vi "FGV Externe Stickstoff Befuellung.vi"(8 "Aktion":T2=enum."Befüllen vorbereiten", 11 "Stiskstoff Befüllzeiten":T1) -> (0 "Ausgang":bool, 1 "Befülldauer":sgl, 2 "Befüllen 2":timestamp, 3 "Befüllen 1":timestamp, 4 "Befüllzeit":dbl, 5 "Timeout":bool, 6 "Aktion":T2=enum."Befüllen vorbereiten")   [LabVIEW 2020, in "Externe Stickstoff Befuellung.lvlib"]
uses:
  Externe Stickstoff Befuellung.lvlib
  Aktionen Externe Stockstoff Befuellung.ctl
  Externe Stickstoff Befuellzeiten.ctl
  Verwaltung/FGV IN Aktionen.ctl
  Konfig-Dateien/FGV Betriebsdaten Aktionen.ctl
  Allgemein/Allgemein.lvlib
  Konfig-Dateien/Konfig-Dateien.lvlib
  Verwaltung/Verwaltung - cRIO.lvlib
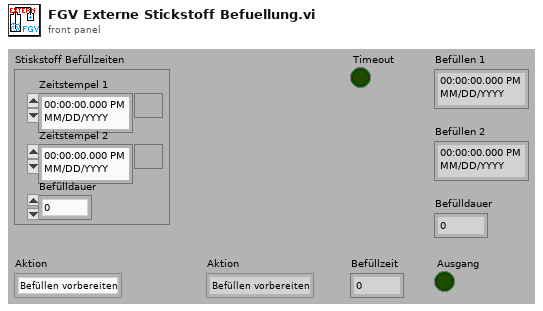
[diagram p1: front panel]
types:
  T1 = typedef "Externe Stickstoff Befuellung.lvlib/Externe Stickstoff Befuellzeiten.ctl" = cluster{"Zeitstempel 1":timestamp, "Zeitstempel 2":timestamp, "Befülldauer":sgl}
  T2 = typedef "Externe Stickstoff Befuellung.lvlib/Aktionen Externe Stockstoff Befuellung.ctl" = enum16{"lesen", "Befüllen vorbereiten", "Befüllen", "Befüllen beenden", "Warten", "deaktiviert", "initialisieren"}
  T3 = typedef "Verwaltung - cRIO.lvlib/FGV IN Aktionen.ctl" = enum16{"lesen", "DI", "AI", "Fühler Br.", "TC", "Fühler Br. TC"}
  T4 = typedef "Konfig-Dateien.lvlib/FGV Betriebsdaten Aktionen.ctl" = enum16{"lesen", "Anlagengrenzw.", "PID Param.", "Sonstige", "Sensor Para."}
  T5 = typedef "Verwaltung - cRIO.lvlib/Digital Eingaenge 0-15.ctl" = cluster{"I0: N2 Nachf. FT-IR voll":bool, "I1: N2 Nachf. Vorrat leer":bool, "I2: (Klimaanlage eingeschaltet)":bool, "I3: (Klimaanlage Störung)":bool, "I4: Trigger Eingang (Messdaten sp.)":bool, "I5: Reserve":bool, "I6: Reserve":bool, "I7: Reserve":bool, "I8: Druckschalter Versorgung ok":bool, "I9: Reserve":bool, "I10: Reserve":bool, "I11: Reserve":bool, "I12: Drucksch. N2 Versorgung":bool, "I13: Reserve":bool, "I14: Drucksch. N2 Optikbox":bool, "I15: (Füllstand Kondensatbehälter)":bool}
  T6 = typedef "Erweiterte Konfig.lvlib/Sonstige Parameter.ctl" = cluster{"Lüfter langsam":sgl, "Lüfter schnell":sgl, "FT-IR Kühlung Soll":sgl, "FT-IR Kühlung Max":sgl, "Überwachung":T7, "Befüllung aktiv":T8, "Stickstoff Befüllzeit":sgl, "Befüllintervall":sgl, "Kalibrierwert FT-IR":sgl, "Offset Ausgang":sgl, "Offset FT-IR":sgl, "Offset Druck FT-IR":sgl, "Dichtheitstest Zeit":sgl, "Dichtheitstest Abfall":sgl, "Dichtheitstest Umfang":T9, "Offset Umgebung":sgl, "Max Taupunkt":sgl, "Pumpendrehzahl":sgl, "ext. Befüllung":T8, "Ext. Stickstoff Befüllzeit":sgl}
  T7 = typedef "Auswahlfeld.ctl" = u16
  T8 = typedef "LogKonfig.lvlib/Auswahlfeld aktiviert-deaktiviert.ctl" = u16
  T9 = typedef "Erweiterte Konfig.lvlib/Dichtheitstest Umfang.ctl" = u16
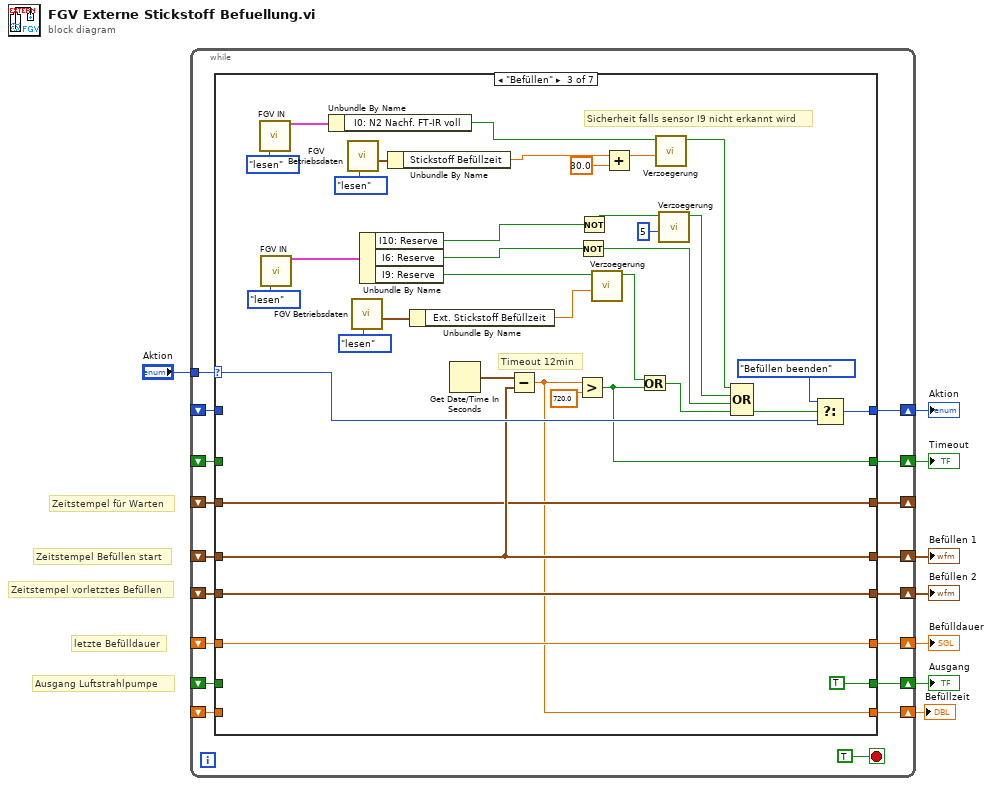
[diagram p0: block diagram]
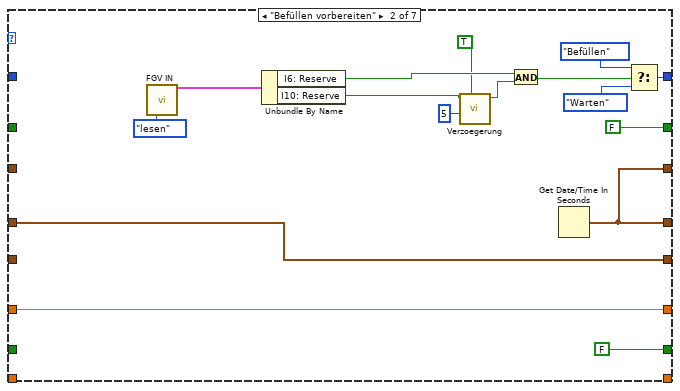
[diagram p3: hidden frame]
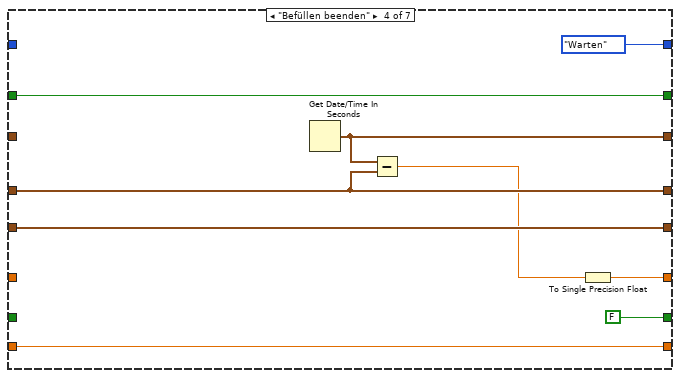
[diagram p4: hidden frame]
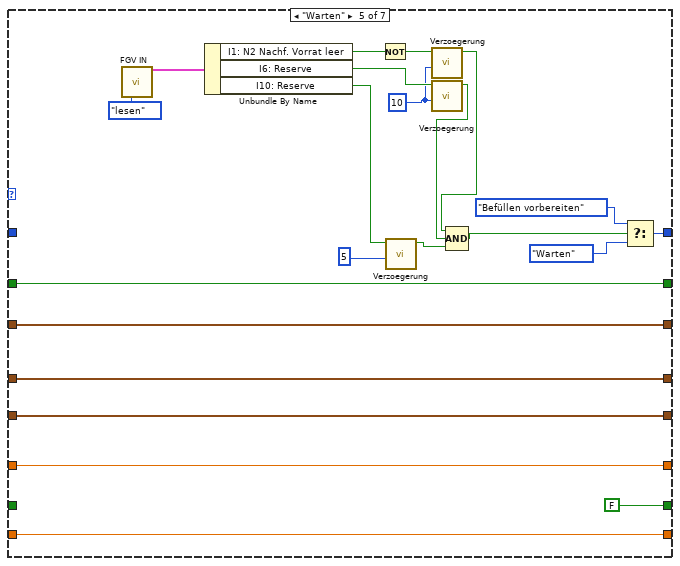
[diagram p5: hidden frame]
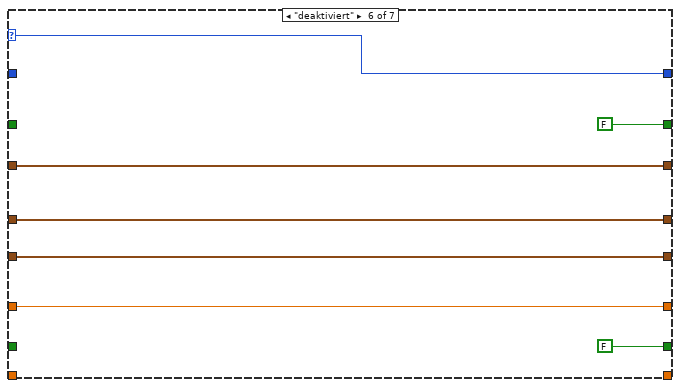
[diagram p6: hidden frame]
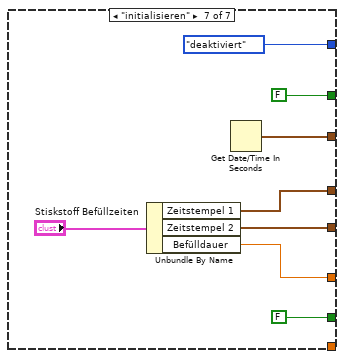
[diagram p7: hidden frame]
diagram:
  # "Zeitstempel für Warten"
  # "Ausgang Luftstrahlpumpe"
  # "Zeitstempel vorletztes Befüllen"
  # "letzte Befülldauer"
  # "Zeitstempel Befüllen start"
  n1 = while {
    tunnel: "Aktion" -> [w23]
    shift-right: [w20] -> w7
    shift-left: _ -> [w18]
    shift-right: [w24] -> w5
    shift-left: _ -> [w16]
    shift-right: [w19] -> w6
    shift-left: _ -> [w17]
    shift-right: [w25] -> w4
    shift-left: _ -> [w15]
    shift-right: [w21] -> w8
    shift-left: _ -> [w14]
    shift-right: [w22] -> w3
    shift-left: _ -> [w13]
    shift-right: [w11] -> _
    shift-left: _ -> [w12]
    shift-right: [w10] -> w1
    shift-left: _ -> [w9]
    stop <- TRUE stop-if-true
    n2 = case shown="\"Befüllen\"" w23 {
      selector: w23 -> [_ _ w84 _ _ w124 _]
      tunnel: [w29 w40 w77 Aktionen_Externe_Stockstoff_Befuellung."Warten" ("Aktion") w111 w124 Aktionen_Externe_Stockstoff_Befuellung."deaktiviert" ("Aktion")] -> w22
      tunnel: [w34 w46 w80 w93 w115 w122 w130] -> w20
      tunnel: [w31 FALSE TRUE FALSE FALSE FALSE FALSE] -> w25
      tunnel: w18 -> [w34 w49 w80 w93 w115 w122 _]
      tunnel: [w32 w48 w81 w88 w112 w120 w131] -> w24
      tunnel: w16 -> [w32 w48 w81 _ w112 w120 _]
      tunnel: [w33 w49 w82 w94 w116 w121 w129] -> w19
      tunnel: w17 -> [w33 _ w82 w94 w116 w121 _]
      tunnel: w15 -> [w31 _ _ _ _ _ _]
      tunnel: [w30 FALSE w74 w91 w109 FALSE FALSE] -> w21
      tunnel: w14 -> [w30 _ _ w91 w109 _ _]
      tunnel: w13 -> [w29 _ _ _ _ _ _]
      tunnel: w12 -> [w28 _ w73 _ w110 w118 _]
      tunnel: [w28 w46 w73 w90 w110 w118 w125] -> w11
      tunnel: [w27 _ w64 w87 w100 _ _] -> w10
      tunnel: w9 -> [w27 _ _ w87 w100 _ _]
      frame "lesen", Default {
      }
      frame "Befüllen vorbereiten" {
        n3 = call "FGV IN.vi"("Aktion"=FGV_IN_Aktionen."lesen") -> ("DI"=w45:T5)  [unwired: 10 in, 4 out]
        n4 = Unbundle By Name(w45) -> ("I6: Reserve"=w41:bool, "I10: Reserve"=w38:bool)
        n5 = call "Verzoegerung.vi"("Abfallverzögerung?"=TRUE, "sec"=u16 5, "Startsignal"=w38) -> ("Zeit abgelaufen?"=w35:bool)  [unwired: 7 in, 1 out]
        n6 = And(x=w41, y=w35) -> (x .and. y?=w39:bool)
        n7 = Get Date/Time In Seconds() -> (seconds since 1Jan1904=w46:timestamp)
        n8 = Select(t=Aktionen_Externe_Stockstoff_Befuellung."Befüllen" ("Aktion"), s=w39, f=Aktionen_Externe_Stockstoff_Befuellung."Warten" ("Aktion")) -> (s? t:f=w40:T2)
      }
      frame "Befüllen" {
        # "Sicherheit falls sensor I9 nicht erkannt wird"
        # "Timeout 12min"
        n9 = call "FGV IN.vi"("Aktion"=FGV_IN_Aktionen."lesen") -> ("DI"=w55:T5)  [unwired: 10 in, 4 out]
        n10 = call "FGV IN.vi"("Aktion"=FGV_IN_Aktionen."lesen") -> ("DI"=w69:T5)  [unwired: 10 in, 4 out]
        n11 = Unbundle By Name(w55) -> ("I0: N2 Nachf. FT-IR voll"=w54:bool)
        n12 = call "FGV Betriebsdaten.vi"("Aktionen"=FGV_Betriebsdaten_Aktionen."lesen") -> ("Sonstige"=w57:T6)  [unwired: 7 in, 3 out]
        n13 = call "FGV Betriebsdaten.vi"("Aktionen"=FGV_Betriebsdaten_Aktionen."lesen") -> ("Sonstige"=w71:T6)  [unwired: 7 in, 3 out]
        n14 = Unbundle By Name(w69) -> ("I10: Reserve"=w63:bool, "I6: Reserve"=w65:bool, "I9: Reserve"=w68:bool)
        n15 = Unbundle By Name(w57) -> ("Stickstoff Befüllzeit"=w59:sgl)
        n16 = Unbundle By Name(w71) -> ("Ext. Stickstoff Befüllzeit"=w86:sgl)
        n17 = Get Date/Time In Seconds() -> (seconds since 1Jan1904=w79:timestamp)
        n18 = Subtract(x=w79, y=w80) -> (x-y=w64:dbl)
        n19 = Greater?(x=w64, y=720.0) -> (0:w74:bool)
        n20 = Not(x=w65) -> (.not. x?=w66:bool)
        n21 = Not(x=w63) -> (.not. x?=w62:bool)
        n22 = call "Verzoegerung.vi"("sec"=w86, "Startsignal"=w68) -> ("Zeit abgelaufen?"=w76:bool)  [unwired: 8 in, 1 out]
        n23 = Add(x=w59, y=sgl 30.0) -> (x+y=w53:sgl)
        n24 = Or(x=w76, y=w74) -> (x .or. y?=w75:bool)
        n25 = call "Verzoegerung.vi"("sec"=w53, "Startsignal"=w54) -> ("Zeit abgelaufen?"=w51:bool)  [unwired: 8 in, 1 out]
        n26 = call "Verzoegerung.vi"("sec"=u16 5, "Startsignal"=w62) -> ("Zeit abgelaufen?"=w61:bool)  [unwired: 8 in, 1 out]
        n27 = Compound Arithmetic op=OR ("Mehrfacharithmetik")(w51, w61, w66, w75) -> (w67:bool)
        n28 = Select(t=Aktionen_Externe_Stockstoff_Befuellung."Befüllen beenden", s=w67, f=w84) -> (s? t:f=w77:T2)
      }
      frame "Befüllen beenden" {
        n29 = Get Date/Time In Seconds() -> (seconds since 1Jan1904=w90:timestamp)
        n30 = Subtract(x=w90, y=w93) -> (x-y=w89:dbl)
        n31 = To Single Precision Float(number=w89) -> (single precision float=w88:sgl)
      }
      frame "Warten" {
        w97 = u16 10 ("sec")
        n32 = call "FGV IN.vi"("Aktion"=FGV_IN_Aktionen."lesen") -> ("DI"=w108:T5)  [unwired: 10 in, 4 out]
        n33 = Unbundle By Name(w108) -> ("I1: N2 Nachf. Vorrat leer"=w107:bool, "I6: Reserve"=w105:bool, "I10: Reserve"=w99:bool)
        n34 = Not(x=w107) -> (.not. x?=w106:bool)
        n35 = call "Verzoegerung.vi"("sec"=u16 5, "Startsignal"=w99) -> ("Zeit abgelaufen?"=w98:bool)  [unwired: 8 in, 1 out]
        n36 = call "Verzoegerung.vi"("sec"=w97, "Startsignal"=w106) -> ("Zeit abgelaufen?"=w104:bool)  [unwired: 8 in, 1 out]
        n37 = call "Verzoegerung.vi"("sec"=w97, "Startsignal"=w105) -> ("Zeit abgelaufen?"=w103:bool)  [unwired: 8 in, 1 out]
        n38 = Compound Arithmetic op=AND ("Mehrfacharithmetik")(w104, w103, w98) -> (w102:bool)
        n39 = Select(t=Aktionen_Externe_Stockstoff_Befuellung."Befüllen vorbereiten" ("Aktion"), s=w102, f=Aktionen_Externe_Stockstoff_Befuellung."Warten") -> (s? t:f=w111:T2)
      }
      frame "deaktiviert" {
      }
      frame "initialisieren" {
        n40 = Unbundle By Name("Stiskstoff Befüllzeiten") -> ("Zeitstempel 1"=w130:timestamp, "Zeitstempel 2"=w129:timestamp, "Befülldauer"=w131:sgl)
        n41 = Get Date/Time In Seconds() -> (seconds since 1Jan1904=w125:timestamp)
      }
    }
  }
  "Aktion" <- w3
  "Timeout" <- w8
  "Befüllen 1" <- w7
  "Befüllen 2" <- w6
  "Befülldauer" <- w5
  "Ausgang" <- w4
  "Befüllzeit" <- w1
